vi "TCP-64b.vi"() -> ()   [LabVIEW 2020]
doc: "创建一个命名服务并在第一个可用端口侦听。当客户端连接该服务时，将发送一个响应字符串至客户端。"
panel:
  out "波形图表 3":i32[](graph)
  in  "停止":bool
  # "概述：演示使用TCP函数初始化可向客户端VI发送数据的命名TCP服务。\n操作步骤:\n1.运行VI。\n2.打开TCP Named Service - Client.vi并按照前面板上的说明操作。\n3.单击停止 停止VI运行。"
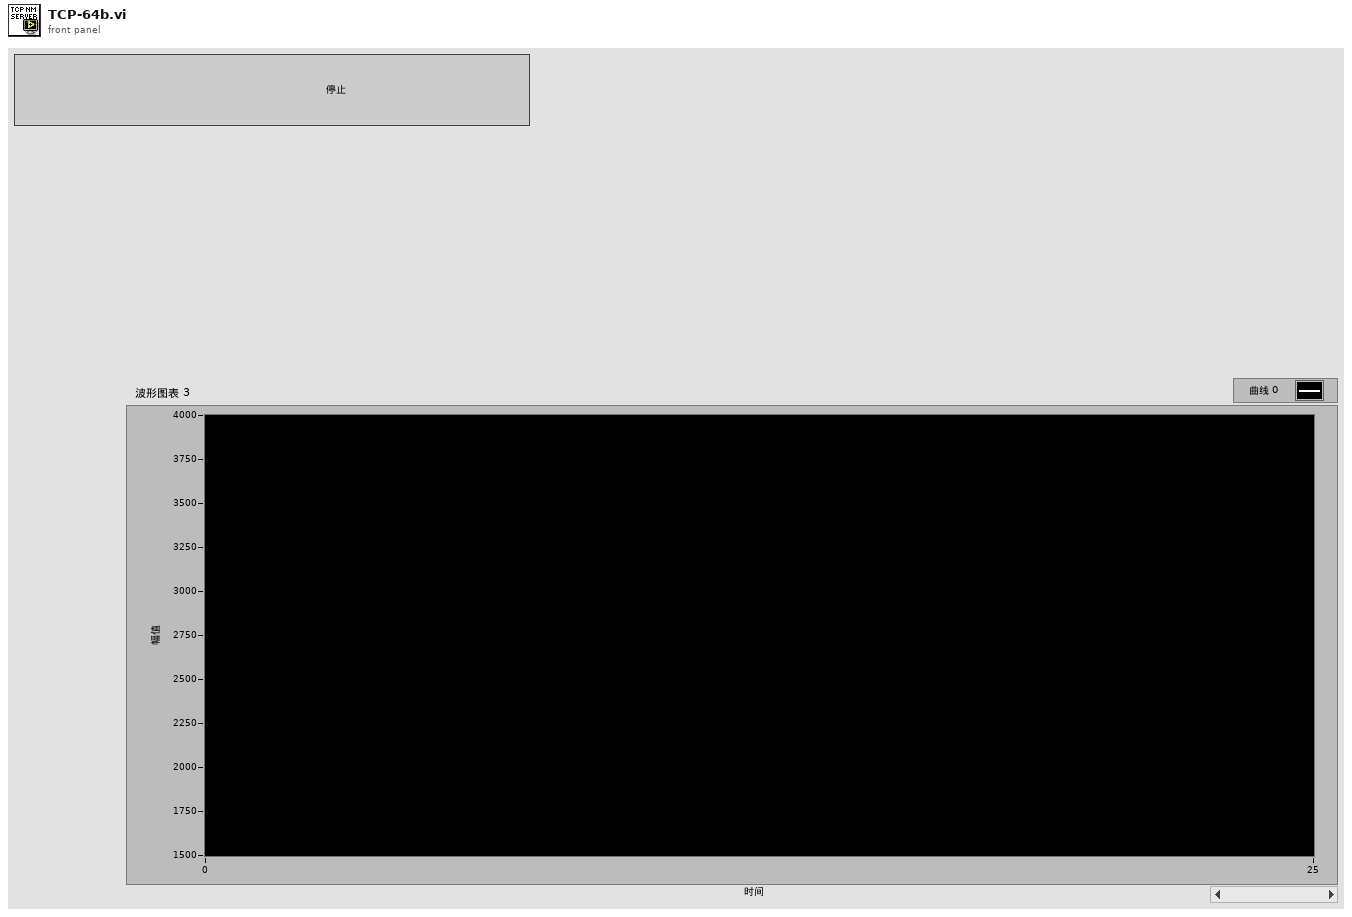
[diagram p1: front panel]
types:
  T1 = enum16{"open", "open or create", "create or replace", "create", "open (read-only)"}
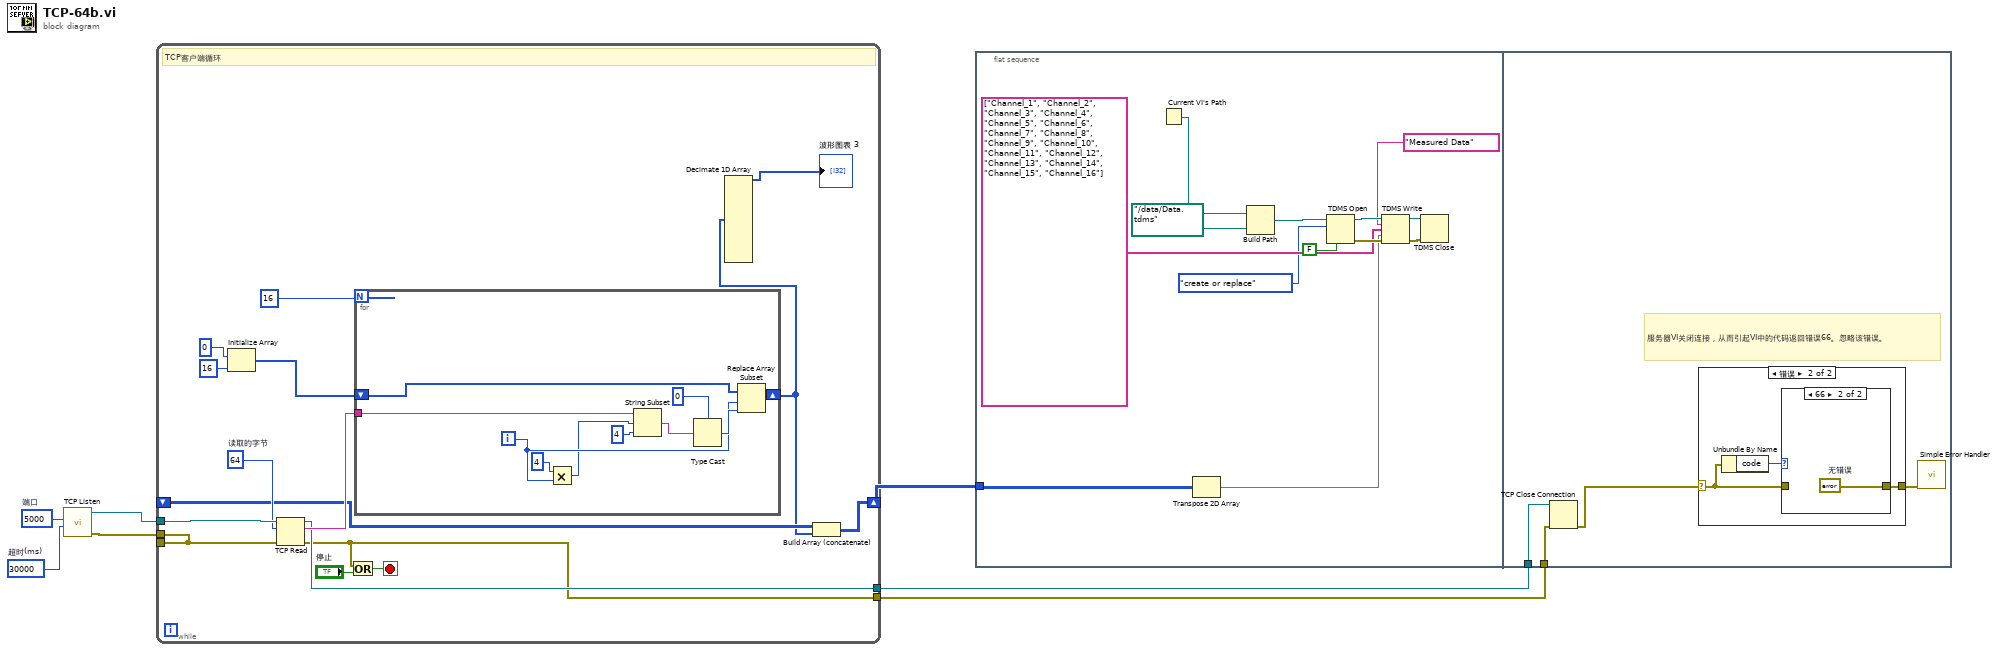
[diagram p0: block diagram]
diagram:
  w6 = u16 5000  # 端口
  w7 = 30000  # 超时(ms)
  n1 = call <vilib>:"TCP Listen.vi"("timeout ms (wait forever: -1)"=w7, "port"=w6) -> ("error out"=w4:errorcluster, "connection ID"=w5:refnum<k5>)  [unwired: 5 in, 3 out]
  n2 = while {
    tunnel: [w20] -> _
    tunnel: w5 -> [w23]
    tunnel: w4 -> [w20]
    shift-right: [w13] -> w3
    shift-left: _ -> [w12]
    tunnel: [w11] -> w2
    tunnel: [w10] -> w1
    stop <- w21 stop-if-true
    w19 = 64  # 读取的字节
    # "TCP客户端循环"
    n3 = Initialize Array(0, 16) -> (w14:i32[])
    n4 = TCP Read(connection ID=w23, bytes to read=w19, error in (no error)=w20) -> (connection ID out=w11:refnum<k5>, data out=w17:string, error out=w10:errorcluster)  [unwired: 2 in]
    n5 = Or(x=w10, y="停止") -> (x .or. y?=w21:bool)
    n6 = for {
      N: u8 16 -> [_]
      shift-right: [w26] -> w8
      shift-left: w14 -> [w27]
      tunnel: w17 -> [w24]
      i -> [w28]
      n7 = Multiply(x=i8 4, y=w28) -> (x*y=w25:i32)
      n8 = String Subset(string=w24, offset (0)=w25, length (rest)=i8 4) -> (substring=w33:string)
      n9 = Type Cast(type=0, x=w33) -> (*(type *) &x=w29:i32)
      n10 = Replace Array Subset(array=w27, new element=w29, index=w28) -> (w26:i32[])
    }
    n11 = Decimate 1D Array(w8) -> (→"波形图表 3":i32[])  [unwired: 11 out]
    n12 = Build Array (concatenate)(w12, w8) -> (w13:i32[][])
  }
  n13 = flat-sequence {
    tunnel: w3 -> [w35]
    tunnel: w2 -> [w48]
    tunnel: w1 -> [w47]
    frame #0 {
      n14 = Current VI's Path() -> (path=w36:path)
      n15 = Transpose 2D Array(2D array=w35) -> (transposed array=w34:i32[][])
      n16 = Build Path(base path=w36, name or relative path=path "../data/Data.tdms" ("file path")) -> (appended path=w42:path)
      n17 = TDMS Open(6:FALSE ("disable buffering (T)"), 10:T1."create or replace" ("operation"), 11:w42) -> (0:w46:errorcluster, 3:w43:refnum<k34>)  [unwired: 4 in]
      n18 = TDMS Write(0:w43, 5:"Measured Data" ("group name"), 7:string[] ["Channel_1", "Channel_2", "Channel_3", "Channel_4", "Channel_5", "Channel_6", "Channel_7", "Channel_8", "Channel_9", "Channel_10", "Channel_11", "Channel_12", "Channel_13", "Channel_14", "Channel_15", "Channel_16"] ("channel names"), 9:w34, 11:w46) -> (4:w44:refnum<k34>, 15:w45:errorcluster)  [unwired: 1 in, 2 out]
      n19 = TDMS Close(8:w45, 11:w44) -> ()  [unwired: 2 out]
    }
    frame #1 {
      # "服务器VI关闭连接，从而引起VI中的代码返回错误66。忽略该错误。"
      n20 = TCP Close Connection(connection ID=w48, error in (no error)=w47) -> (error out=w49:errorcluster)  [unwired: 1 in, 1 out]
      n21 = case shown="错误" w49 {
        selector: w49 -> [w51 w53]
        tunnel: [w51 w52] -> w50
        frame No Error {
        }
        frame Error {
          n22 = Unbundle By Name(w53) -> ("code"=w54:i32)
          n23 = case shown="66" w54 {
            tunnel: w53 -> [w55 _]
            tunnel: [w55 w56] -> w52
            frame Default {
            }
            frame 66 {
              w56 = errorcluster {"status"=FALSE, "code"=0, "source"=""}  # 无错误
            }
          }
        }
      }
      n24 = call <vilib>:"Simple Error Handler.vi"("error in (no error)"=w50) -> ()  [unwired: 4 in, 5 out]
    }
  }
